vi "tm3samp_acquirereplay.vi"() -> ()   [LabVIEW 2012]
panel:
  out "Image":u16[][](graph)
  in  "Play":bool
  in  "Acquire":bool
  out "Current Frame Index":i32=-1
  in  "Frames to Capture":i32=100
  out "Camera Serial":string
  out "Camera Model":string
  out "Camera Version":string
  out "Total Frames":i32
  out "error out":errorcluster
  in  "quit":bool
  # "This is an example of how to capture\ndata at full speed to RAM, then read \nthe data from the buffer later."
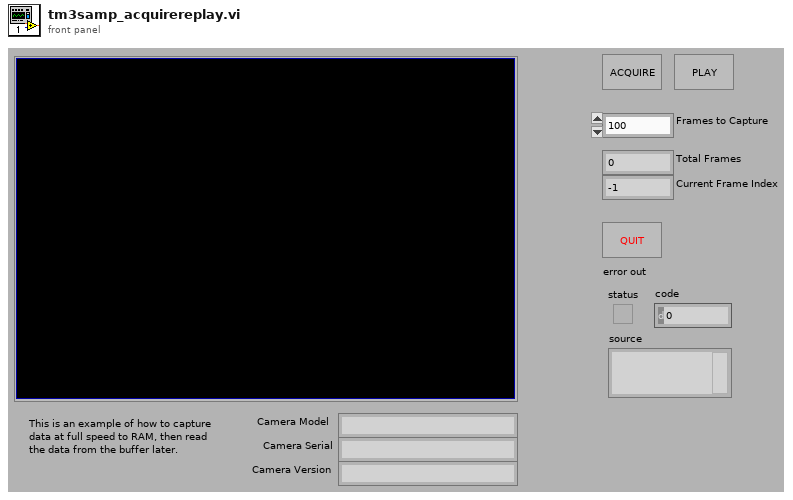
[diagram p1: front panel]
types:
  T1 = cluster{"width":u32, "height":u32, "datatype":u32}
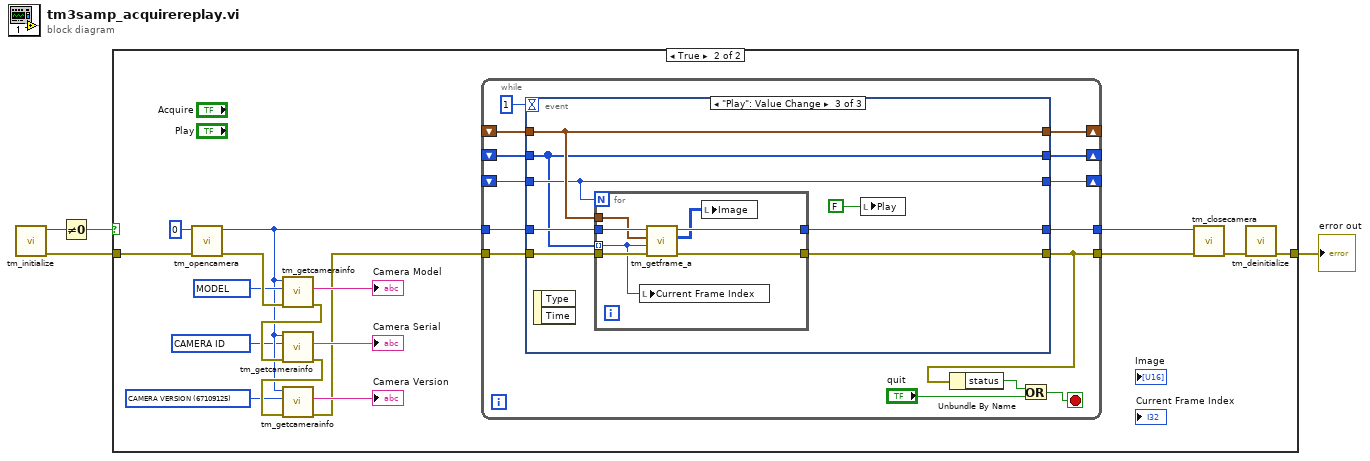
[diagram p0: block diagram]
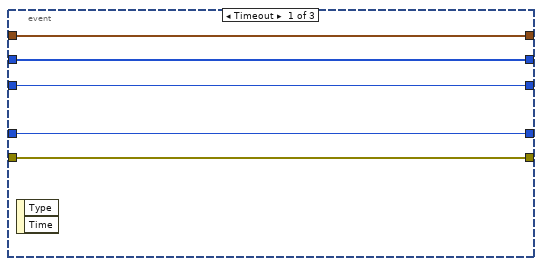
[diagram p3: hidden frame]
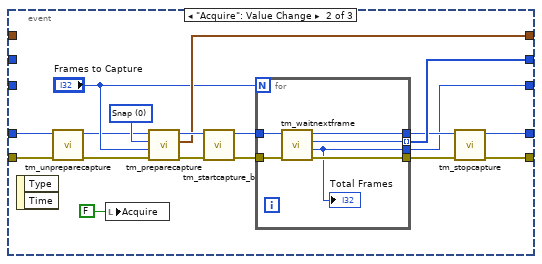
[diagram p4: hidden frame]
diagram:
  n1 = call <userlib>:"tm_initialize.vi"() -> ("error out"=w1:errorcluster, "Number Of Cameras"=w2:u32)  [unwired: 10 in]
  n2 = Not Equal To 0?(x=w2) -> (x != 0?=w4:bool)
  n3 = case shown="True" w4 {
    tunnel: [w5 w19] -> w3
    tunnel: w1 -> [w5 w22]
    frame False {
    }
    frame True {
      w6 = u32 67109122 items=["BUS"=67109121, "CAMERA ID"=67109122, "VENDOR"=67109123, "MODEL"=67109124, "CAMERA VERSION"=67109125, "DRIVER VERSION"=67109126, "MODULE VERSIOIN"=67109127, "DCAMAPI VERSION"=67109128] ("Info ID")
      w14 = u32 67109125 items=["BUS"=67109121, "CAMERA"=67109122, "VENDOR"=67109123, "MODEL"=67109124, "CAMERA VERSION"=67109125, "DRIVER VERSION"=67109126, "MODULE VERSIOIN"=67109127, "DCAMAPI VERSION"=67109128] ("Info ID")
      w17 = u32 67109124 items=["BUS"=67109121, "CAMERA"=67109122, "VENDOR"=67109123, "MODEL"=67109124, "CAMERA VERSION"=67109125, "DRIVER VERSION"=67109126, "MODULE VERSIOIN"=67109127, "DCAMAPI VERSION"=67109128] ("Info ID")
      n4 = call <userlib>:"tm_opencamera.vi"("error in (no error)"=w22, "Camera Index"=u32 0) -> ("error out"=w18:errorcluster, "Handle out"=w10:u32)  [unwired: 8 in]
      n5 = call <userlib>:"tm_getcamerainfo.vi"("error in (no error)"=w18, "Info ID"=w17, "Handle in"=w10) -> ("error out"=w16:errorcluster, "String"=→"Camera Model":string)  [unwired: 6 in, 1 out]
      n6 = call <userlib>:"tm_getcamerainfo.vi"("error in (no error)"=w16, "Info ID"=w6, "Handle in"=w10) -> ("error out"=w15:errorcluster, "String"=→"Camera Serial":string)  [unwired: 6 in, 1 out]
      n7 = call <userlib>:"tm_getcamerainfo.vi"("error in (no error)"=w15, "Info ID"=w14, "Handle in"=w10) -> ("error out"=w9:errorcluster, "String"=→"Camera Version":string)  [unwired: 6 in, 1 out]
      n8 = while {
        tunnel: [w27] -> w8
        tunnel: [w36] -> w7
        tunnel: w10 -> [w34]
        tunnel: w9 -> [w33]
        shift-right: [w23] -> _
        shift-left: _ -> [w30]
        shift-right: [w32] -> _
        shift-left: _ -> [w31]
        shift-right: [w29] -> _
        shift-left: _ -> [w28]
        stop <- w24 stop-if-true
        n9 = event shown="[2] \"Play\": Value Change" {
          selector: _ -> [_ _ _]
          dyn-events: _ -> [_ _ _]
          timeout: 1 -> [_ _ _]
          tunnel: [w40 w49 w73] -> w36
          tunnel: [w41 w50 w72] -> w27
          tunnel: w33 -> [w41 w45 w69]
          tunnel: w34 -> [w40 w42 w70]
          tunnel: [w39 w54 w71] -> w32
          tunnel: w31 -> [w39 _ w71]
          tunnel: [w37 w46 w68] -> w23
          tunnel: w30 -> [w37 _ w68]
          tunnel: [w38 w53 w66] -> w29
          tunnel: w28 -> [w38 _ w66]
          event Timeout {
            n10 = event-data() -> ()  [unwired: 1 in, 2 out]
          }
          event "Acquire": Value Change {
            w55 = 0 items=["Snap", "Sequence"] ("Capture mode")
            n11 = event-data() -> ()  [unwired: 1 in, 2 out]
            n12 = call <userlib>:"tm_unpreparecapture.vi"("error in (no error)"=w45, "Handle in"=w42) -> ("error out"=w44:errorcluster, "Handle out"=w43:u32)  [unwired: 8 in]
            n13 = local write "Acquire"(FALSE) -> ()
            n14 = call <userlib>:"tm_preparecapture.vi"("error in (no error)"=w44, "Frames"="Frames to Capture", "Capture mode"=w55, "Handle in"=w43) -> ("error out"=w56:errorcluster, "Buffer"=w54:T1, "Handle out"=w57:u32)  [unwired: 4 in, 1 out]
            n15 = call <userlib>:"tm_startcapture_b.vi"("error in (no error)"=w56, "Handle in"=w57) -> ("error out"=w58:errorcluster, "Handle out"=w59:u32)  [unwired: 8 in]
            n16 = for {
              N: "Frames to Capture" -> [_]
              tunnel: w58 -> [w64]
              tunnel: w59 -> [w65]
              tunnel: [w62] -> w53 mode=indexing
              tunnel: [w63] -> w48
              tunnel: [w60] -> w46
              tunnel: [w61] -> w47
              n17 = call <userlib>:"tm_waitnextframe.vi"("error in (no error)"=w64, "Handle in"=w65) -> ("error out"=w61:errorcluster, "Frame Count"=w60:i32, "Frame Index"=w62:i32, "Handle out"=w63:u32)  [unwired: 6 in]
              "Total Frames" <- w60
            }
            n18 = call <userlib>:"tm_stopcapture.vi"("error in (no error)"=w47, "Handle in"=w48) -> ("error out"=w50:errorcluster, "Handle out"=w49:u32)  [unwired: 8 in]
          }
          event "Play": Value Change {
            n19 = event-data() -> ()  [unwired: 1 in, 2 out]
            n20 = for {
              N: w68 -> [_]
              tunnel: w66 -> [w75] mode=indexing
              tunnel: w69 -> [w80]
              tunnel: w70 -> [w79]
              tunnel: w71 -> [w74]
              tunnel: [w78] -> w72
              tunnel: [w77] -> w73
              n21 = local write "Current Frame Index"(w75) -> ()
              n22 = call <userlib>:"tm_getframe_a.vi"("error in (no error)"=w80, "Frame Index"=w75, "Buffer"=w74, "Handle in"=w79) -> ("error out"=w78:errorcluster, "Data 16"=w76:u16[][], "Handle out"=w77:u32)  [unwired: 3 in, 2 out]
              n23 = local write "Image"(w76) -> ()
            }
            n24 = local write "Play"(FALSE) -> ()
          }
        }
        n25 = Unbundle By Name(w27) -> ("status"=w26:bool)
        n26 = Or(x=w26, y="quit") -> (x .or. y?=w24:bool)
      }
      n27 = call <userlib>:"tm_closecamera.vi"("error in (no error)"=w8, "Handle in"=w7) -> ("error out"=w20:errorcluster)  [unwired: 9 in]
      n28 = call <userlib>:"tm_deinitialize.vi"("error in (no error)"=w20) -> ("error out"=w19:errorcluster)  [unwired: 10 in]
    }
  }
  "error out" <- w3
